vi "Warm Laser.vi"(8 "error in (no error)":errorcluster, 11 "Laser Controller API in":refnum<class "Laser Controller.lvclass">) -> (0 "error out":errorcluster, 3 "Laser Controller API out":refnum<class "Laser Controller.lvclass">)   [LabVIEW 2022 SP3, in "Laser Controller.lvclass"]
uses:
  Laser Controller.lvclass
  Laser Controller.lvclass/Laser Controller.ctl
  Laser State Data/Laser State Data.lvclass/Laser State Data.ctl
  Laser State Data/Laser State.ctl
  Laser State Data/Write Laser State.vi
  Laser State Data/Read Laser State.vi
  Laser Process/Laser Process Messages/Warm Laser Msg/Warm Laser Msg.lvclass
  C:/Program Files/National Instruments/LabVIEW 2022/vi.lib/ActorFramework/Message/Message.lvclass
  <vilib>/Utility/error.llb/Error Cluster From Error Code.vi
  <vilib>/ErrorRing/Error Ring.xnode
  XY Stage/Process Actor/Process Framework/Interlock Q Class/Interlock Q Class.lvclass
  Laser State Data/Laser State Data.lvclass
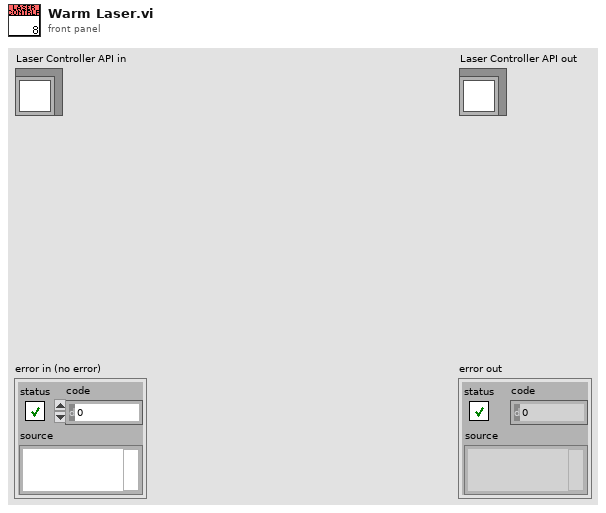
[diagram p1: front panel]
types:
  T1 = typedef "Laser State Data.lvclass/Laser State.ctl" = enum16{"Idle", "Warming", "Ready", "Firing"}
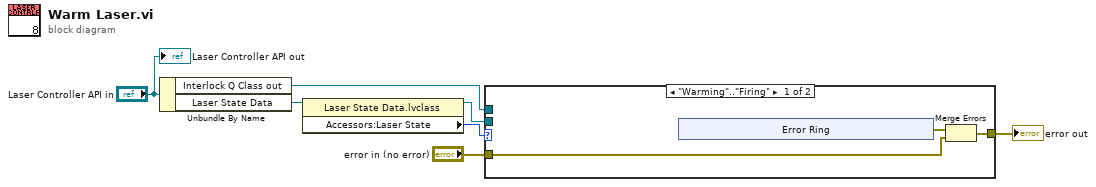
[diagram p0: block diagram]
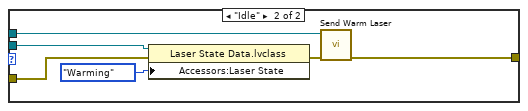
[diagram p2: hidden frame]
diagram:
  n1 = Unbundle By Name("Laser Controller API in") -> ("Interlock Q Class out"=w6:refnum<class "Interlock Q Class.lvclass">, "Laser State Data"=w3:refnum<data-value>)
  n2 = property class="Laser State Data.lvclass"(reference=w3) -> (reference out=w1:refnum<data-value>, "Accessors:Laser State"=w2:T1)  [unwired: 1 in, 1 out]
  n3 = case shown="\"Warming\"..\"Firing\"" w2 {
    tunnel: w6 -> [_ w21]
    tunnel: "error in (no error)" -> [w9 w16]
    tunnel: [w8 w20] -> w4
    tunnel: w1 -> [_ w19]
    frame "Warming".."Firing" {
      n4 = xnode "Error Ring"() -> ("error out"=w10:errorcluster)
      n5 = Merge Errors(w10, w9) -> (w8:errorcluster)
    }
    frame "Idle" {
      n6 = property class="Laser State Data.lvclass"(reference=w19, error in=w16, "Accessors:Laser State"=Laser_State."Warming" ("Laser State")) -> (error out=w17:errorcluster)  [unwired: 1 out]
      n7 = call "Send Warm Laser.vi"("error in (no error)"=w17, "Interlock Q Class in"=w21) -> ("error out"=w20:errorcluster)  [unwired: 8 in, 1 out]
    }
  }
  "error out" <- w4
  "Laser Controller API out" <- "Laser Controller API in"
